vi "Write Test Type.vi"(10 "Test Type":string, 11 "Test in":refnum<class "Test.lvclass">) -> (3 "Test out":refnum<class "Test.lvclass">)   [LabVIEW 2018, in "Test.lvclass"]
uses:
  Test.lvclass
  Test.lvclass/Test.ctl
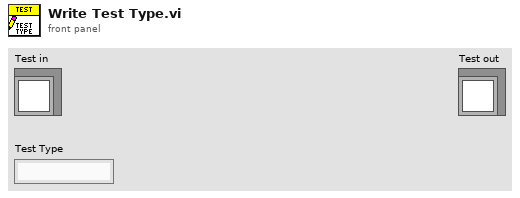
[diagram p1: front panel]
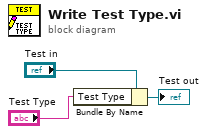
[diagram p0: block diagram]
diagram:
  n1 = Bundle By Name(cluster="Test in", "Test Type"="Test Type") -> (→"Test out":refnum<class "Test.lvclass">)
